vi "Real Daq Send.vi"(8 "error in (no error)":errorcluster, 9 "LBCB Select":T1, 10 "Commands":dbl[](array[numeric]), 11 "Daq Actions":T2) -> (0 "error out":errorcluster)   [LabVIEW 2009]
uses:
  Daq Actions.ctl
  Data Access Objects/Metadata/LBCB Number.ctl
  Data Access Objects/Metadata/Persistant DAO Actions.ctl
  Data Access Objects/Metadata/LBCB Filter.ctl
  <vilib>/DAQmx/write.llb/DAQmx Write (Analog 1D DBL NChan 1Samp).vi
panel:
  out "Channels":refnum<k21>
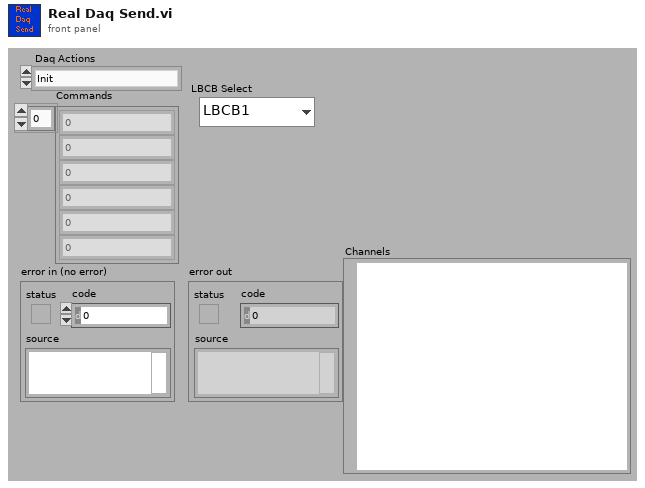
[diagram p1: front panel]
types:
  T1 = typedef "LBCB Number.ctl" = enum16{"LBCB1", "LBCB2"}
  T2 = typedef "Daq Actions.ctl" = enum16{"Init", "Send Commands", "Get Responses", "Stop"}
  T3 = typedef "Persistant DAO Actions.ctl" = enum16{"Init", "Get", "Set", "Load", "Save"}
  T4 = typedef "LBCB Filter.ctl" = enum16{"LBCB 1", "LBCB 2", "Both"}
  T5 = typedef "Number Of LBCBs.ctl" = enum16{"1", "2"}
  T6 = typedef "Actuator Channel Names.ctl" = cluster{"X1":refnum<k21>, "X2":refnum<k21>, "Y1":refnum<k21>, "Z1":refnum<k21>, "Z2":refnum<k21>, "Z3":refnum<k21>}
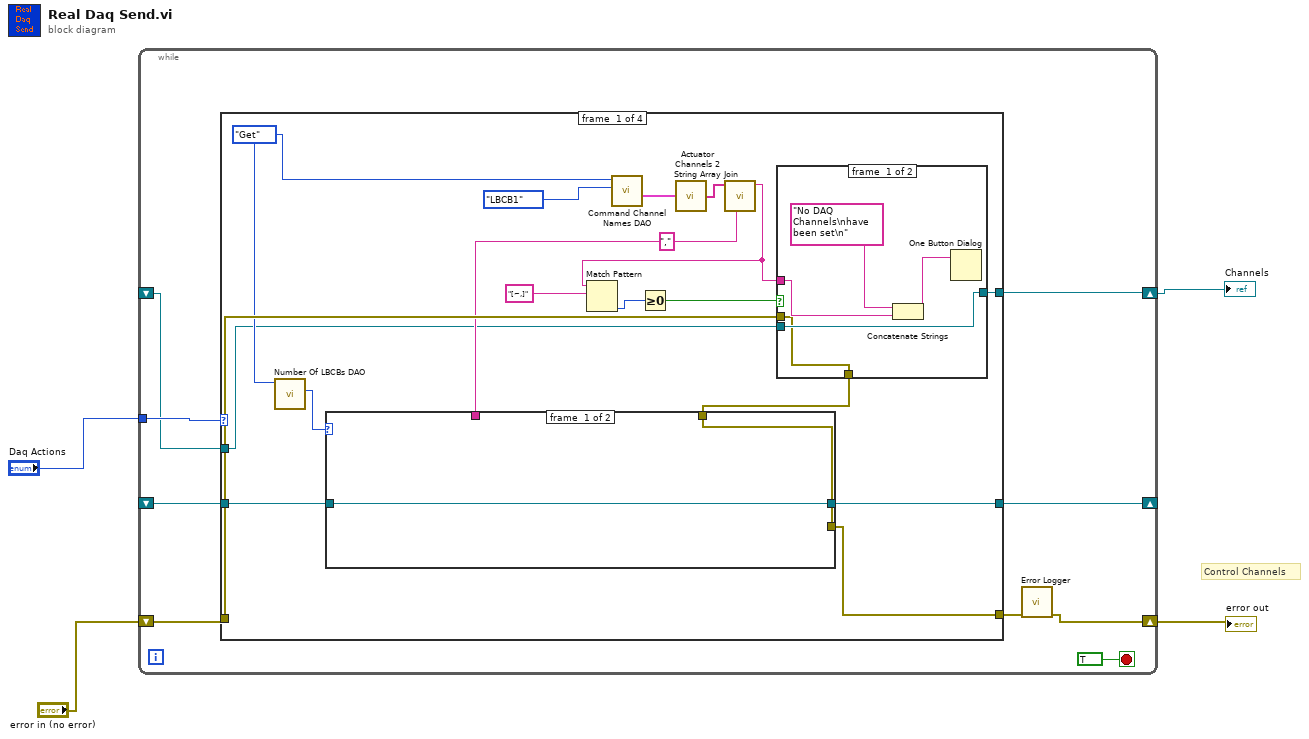
[diagram p0: block diagram]
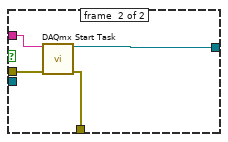
[diagram p2: hidden frame]
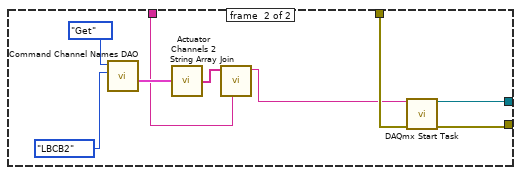
[diagram p3: hidden frame]
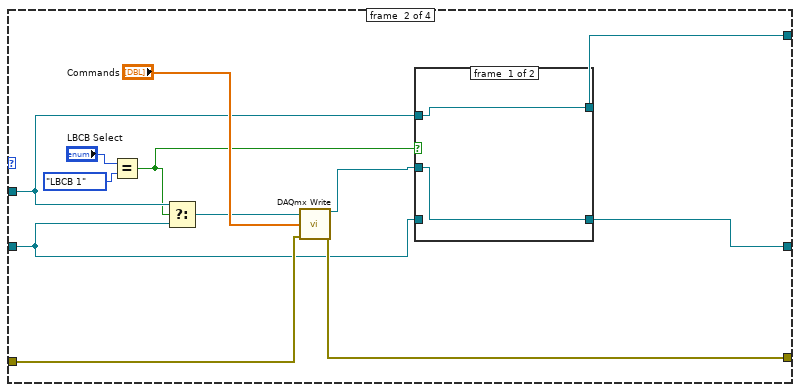
[diagram p4: hidden frame]
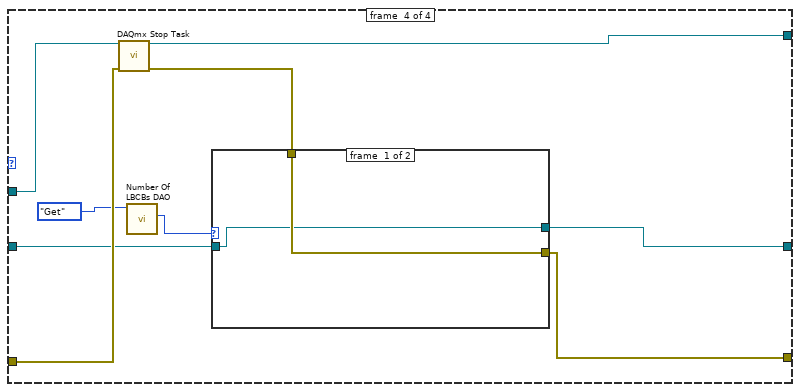
[diagram p7: hidden frame]
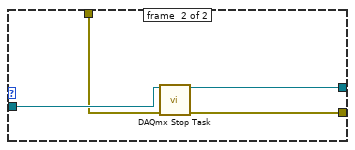
[diagram p8: hidden frame]
diagram:
  # "Control Channels"
  n1 = while {
    tunnel: "Daq Actions" -> [w13]
    shift-right: [w11] -> w1
    shift-left: _ -> [w10]
    shift-right: [w8] -> w2
    shift-left: "error in (no error)" -> [w9]
    shift-right: [w6] -> _
    shift-left: _ -> [w5]
    stop <- TRUE stop-if-true
    n2 = case shown="\"Init\"" w13 {
      tunnel: [w30 w57 w69 w78] -> w11
      tunnel: w10 -> [w14 w54 w69 w77]
      tunnel: w9 -> [w29 w61 w68 w76]
      tunnel: [w27 w60 w68 w73] -> w7
      tunnel: [w26 w55 w67 w72] -> w6
      tunnel: w5 -> [w25 w56 w67 w75]
      frame #0 {
        w20 = Persistant_DAO_Actions."Get" ("Actions")
        w21 = "," ("delimiter")
        n3 = call "Number Of LBCBs DAO.vi"("Actions"=w20) -> ("Number of\nLBCBs Out"=w19:T5)  [unwired: 4 in, 6 out]
        n4 = call "Command Channel Names DAO.vi"("LBCB Number"=LBCB_Number."LBCB1", "Actions"=w20) -> ("Names Out"=w23:T6)  [unwired: 3 in, 6 out]
        n5 = call "Actuator Channels 2 String Array.vi"("Actuator Channels"=w23) -> ("Array"=w22:string[])
        n6 = call "Join.vi"("delimiter"=w21, "Array"=w22) -> ("Joined Result"=w15:string)  [unwired: 9 out]
        n7 = Match Pattern(string=w15, regular expression="[~,]") -> (offset past match=w17:i32)  [unwired: 4 out]
        n8 = Greater Or Equal To 0?(x=w17) -> (x >= 0?=w16:bool)
        n9 = case shown="False" w16 {
          tunnel: [w32 w39] -> w30
          tunnel: w29 -> [w31 w38]
          tunnel: [w31 w37] -> w28
          tunnel: w15 -> [w33 w36]
          tunnel: w14 -> [w32 _]
          frame #0 {
            n10 = Concatenate Strings("No DAQ Channels\nhave been set\n" ("string"), w33) -> (w34:string)
            n11 = One Button Dialog(message=w34) -> ()  [unwired: 2 out]
          }
          frame #1 {
            n12 = call <vilib>:"DAQmx Start Task.vi"("task/channels in"=w36, "error in"=w38) -> ("task out"=w39:refnum<k21>, "error out"=w37:errorcluster)  [unwired: 12 out]
          }
        }
        n13 = case shown="\"2\"" w19 {
          tunnel: w28 -> [w41 w50]
          tunnel: [w41 w49] -> w27
          tunnel: [w40 w48] -> w26
          tunnel: w25 -> [w40 _]
          tunnel: w21 -> [_ w44]
          frame #0 {
          }
          frame #1 {
            n14 = call "Command Channel Names DAO.vi"("LBCB Number"=LBCB_Number."LBCB2", "Actions"=Persistant_DAO_Actions."Get") -> ("Names Out"=w46:T6)  [unwired: 3 in, 6 out]
            n15 = call "Actuator Channels 2 String Array.vi"("Actuator Channels"=w46) -> ("Array"=w47:string[])
            n16 = call "Join.vi"("delimiter"=w44, "Array"=w47) -> ("Joined Result"=w43:string)  [unwired: 9 out]
            n17 = call <vilib>:"DAQmx Start Task.vi"("task/channels in"=w43, "error in"=w50) -> ("task out"=w48:refnum<k21>, "error out"=w49:errorcluster)  [unwired: 12 out]
          }
        }
      }
      frame #1 {
        n18 = Equal?(x="LBCB Select", y=LBCB_Filter."LBCB 1" ("LBCB Filter")) -> (x = y?=w51:bool)
        n19 = Select(t=w54, s=w51, f=w56) -> (s? t:f=w59:refnum<k21>)
        n20 = call-poly <vilib>:"DAQmx Write.vi"("task/channels in"=w59, "data"="Commands", "error in"=w61) -> ("task out"=w58:refnum<k21>, "error out"=w60:errorcluster)  [unwired: 2 in, 9 out]
        n21 = case shown="False" w51 {
          tunnel: w58 -> [w63 w66]
          tunnel: [w64 w66] -> w57
          tunnel: w56 -> [_ w65]
          tunnel: [w63 w65] -> w55
          tunnel: w54 -> [w64 _]
          frame #0 {
          }
          frame #1 {
          }
        }
      }
      frame #2 {
      }
      frame #3 {
        n22 = call <vilib>:"DAQmx Stop Task.vi"("task/channels in"=w77, "error in"=w76) -> ("task out"=w78:refnum<k21>, "error out"=w74:errorcluster)  [unwired: 12 out]
        n23 = call "Number Of LBCBs DAO.vi"("Actions"=Persistant_DAO_Actions."Get") -> ("Number of\nLBCBs Out"=w71:T5)  [unwired: 4 in, 6 out]
        n24 = case shown="\"1\", Default" w71 {
          tunnel: w75 -> [w79 w84]
          tunnel: w74 -> [w80 w83]
          tunnel: [w80 w82] -> w73
          tunnel: [w79 w81] -> w72
          frame #0 {
          }
          frame #1 {
            n25 = call <vilib>:"DAQmx Stop Task.vi"("task/channels in"=w84, "error in"=w83) -> ("task out"=w81:refnum<k21>, "error out"=w82:errorcluster)  [unwired: 12 out]
          }
        }
      }
    }
    n26 = call "Error Logger.vi"("error in (no error)"=w7) -> ("error out"=w8:errorcluster)  [unwired: 1 in, 9 out]
  }
  "error out" <- w2
  "Channels" <- w1
